vi "Receive Auth Response.vi"(8 "error in (no error)":errorcluster, 11 "Connection in":refnum<class "Connection.lvclass">) -> (0 "error out":errorcluster, 1 "timeout":bool, 2 "Response":T1, 3 "Connection out":refnum<class "Connection.lvclass">)   [LabVIEW 2013, in "Connection_GOSPL.lvlib" / "Connection.lvclass"]
uses:
  Connection.lvclass
  auth response -- cluster.ctl
  Connection.lvclass/Connection.ctl
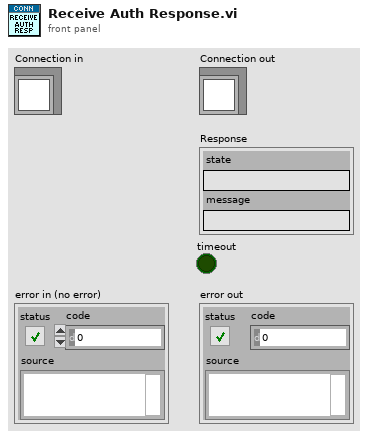
[diagram p1: front panel]
types:
  T1 = typedef "Connection_GOSPL.lvlib/Connection.lvclass/auth response -- cluster.ctl" = cluster{"state":string, "message":string}
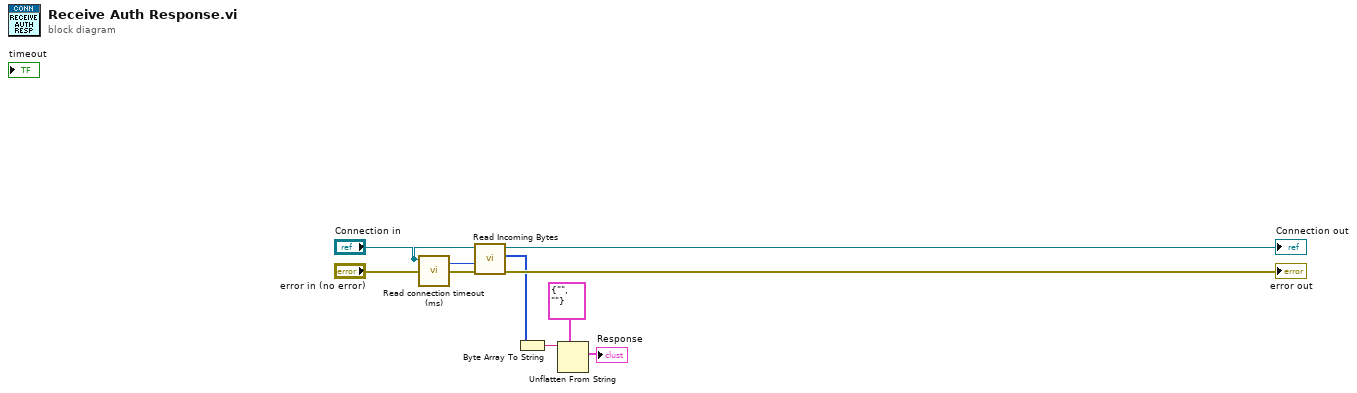
[diagram p0: block diagram]
diagram:
  n1 = call "Read connection timeout (ms).vi"("Connection in"="Connection in") -> ("connection timeout (ms)"=w5:i32)  [unwired: 8 in, 2 out]
  n2 = call-dynamic "Read Incoming Bytes.vi"("error in (no error)"="error in (no error)", "timeout (1000 ms)"=w5, "Connection in"="Connection in") -> ("error out"=→"error out":errorcluster, "Bytes"=w4:u8[], "Connection out"=→"Connection out":refnum<class "Connection.lvclass">)  [unwired: 4 in, 2 out]
  n3 = Byte Array To String(unsigned byte array=w4) -> (string=w1:string)
  n4 = Unflatten From String(type=T1 {"state"="", "message"=""} ("Response"), binary string=w1) -> (value=→"Response":T1)  [unwired: 3 in, 2 out]
